vi "Analytical Inverse Kinematics (6R Type 1).vi"(8 "error in (no error)":errorcluster, 10 "end effector transform":T1, 11 "6R type 1 serial arm in":refnum<class "NI_Robotics_6R Type 1 Serial Arm Class.lvclass">) -> (0 "error out":errorcluster, 1 "number of valid solutions":i32, 2 "joint positions":T1, 3 "6R type 1 serial arm out":refnum<class "NI_Robotics_6R Type 1 Serial Arm Class.lvclass">)   [LabVIEW 2017, in "NI_Robotics_6R Type 1 Serial Arm Class.lvclass"]
doc: "Returns the joint angles of a 6R, 5R, or SCARA arm given the posture of the end effector relative to the arm base. Wire data to the <B>X</B><B>_serial arm in</B> input, where <B>X</B> is the arm type, to determine the polymorphic instance to use or manually select the instance."
uses:
  <vilib>/robotics/Kinematics/Analytical/6R/Type 1/NI_Robotics_6R Type 1 Serial Arm Class.lvclass
  c:/Program Files (x86)/National Instruments/LabVIEW 2017/vi.lib/robotics/Kinematics/Robot/NI_Robotics_Serial Robot Arm.lvclass
  c:/Program Files (x86)/National Instruments/LabVIEW 2017/vi.lib/robotics/Kinematics/Analytical/Generic/NI_Robotics_Analytical Serial Arm Class.lvclass
  <vilib>/Analysis/Matrix/Datatypes/RealMatrix.ctl
  <vilib>/robotics/Kinematics/Link/NI_Robotics_Link.lvclass/NI_Robotics_Link.ctl
  <vilib>/Analysis/baseanly.llb/Real A x B.vi
  <vilib>/robotics/Kinematics/Link/Get Kinematic Parameters.vi
  <vilib>/robotics/Kinematics/Analytical/Generic/NI_Robotics_Analytical Serial Arm Class.lvclass
  <vilib>/robotics/Kinematics/Analytical/Generic/Accessors/Read alpha_n0.vi
  <vilib>/robotics/Kinematics/Robot/Get Links.vi
  <vilib>/Analysis/baseanly.llb/Real Inverse Matrix.vi
  <vilib>/robotics/Kinematics/Robot/NI_Robotics_Serial Robot Arm.lvclass
  <vilib>/Analysis/NI_AALBase.lvlib
  <vilib>/robotics/Kinematics/NI_Kinematics.lvlib
  <vilib>/Analysis/Matrix/NI_Matrix.lvlib
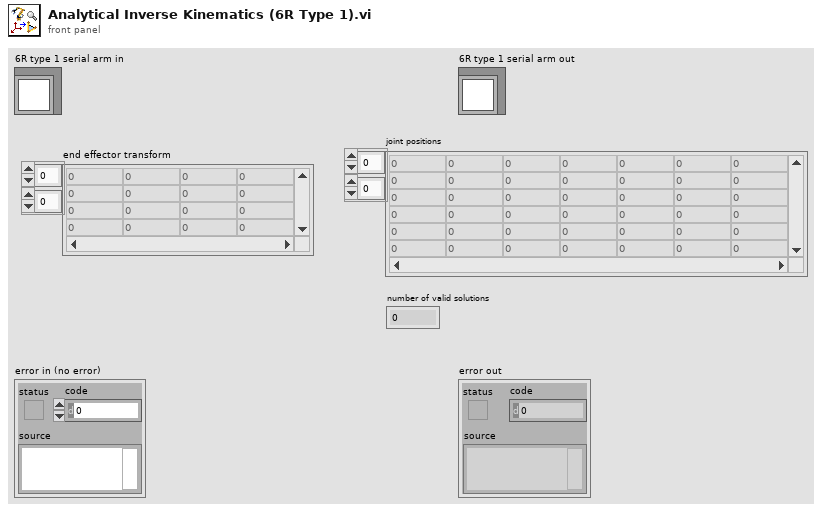
[diagram p1: front panel]
types:
  T1 = typedef "NI_Matrix.lvlib/RealMatrix.ctl" = dbl[][]
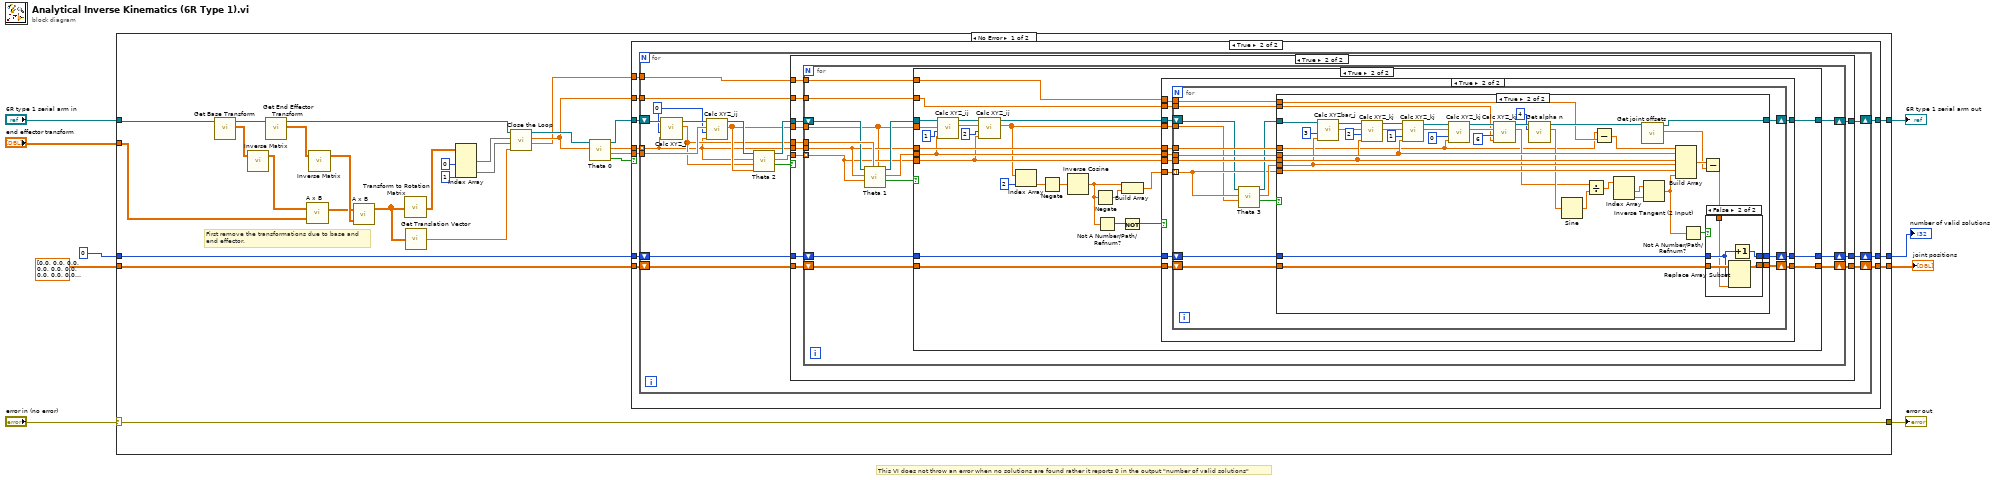
[diagram p0: block diagram]
diagram:
  # "This VI does not throw an error when no solutions are found rather it reports 0 in the output \"number of valid solutions\""
  n1 = case shown="No Error" "error in (no error)" {
    selector: "error in (no error)" -> [w38 w215]
    tunnel: [w38 w215] -> w8
    tunnel: [w27 w214] -> w6
    tunnel: "6R type 1 serial arm in" -> [w18 w214]
    tunnel: "end effector transform" -> [w12 _]
    tunnel: dbl[][] [[0.0, 0.0, 0.0, 0.0, 0.0, 0.0], [0.0, 0.0, 0.0, 0.0, 0.0, 0.0], [0.0, 0.0, 0.0, 0.0, 0.0, 0.0], [0.0, 0.0, 0.0, 0.0, 0.0, 0.0], [0.0, 0.0, 0.0, 0.0, 0.0, 0.0], [0.0, 0.0, 0.0, 0.0, 0.0, 0.0], [0.0, 0.0, 0.0, 0.0, 0.0, 0.0], [0.0, 0.0, 0.0, 0.0, 0.0, 0.0]] ("Solutions") -> [w26 w212]
    tunnel: [w25 w212] -> w1
    tunnel: 0 -> [w24 w213]
    tunnel: [w23 w213] -> w2
    frame No Error {
      # "First remove the transformations due to base and\nend effector."
      n2 = call <vilib>:"Get Base Transform.vi"("serial arm in"=w18) -> ("base transform"=w35:T1, "serial arm out"=w37:refnum<class "NI_Robotics_6R Type 1 Serial Arm Class.lvclass">)  [unwired: 8 in, 1 out]
      n3 = call-poly <vilib>:"Inverse Matrix.vi"("Input Matrix"=w35) -> ("Inverse Matrix"=w13:T1)  [unwired: 1 in, 1 out]
      n4 = call <vilib>:"Get End Effector Transform.vi"("serial arm in"=w37) -> ("end effector transform"=w36:T1, "serial arm out"=w30:refnum<class "NI_Robotics_6R Type 1 Serial Arm Class.lvclass">)  [unwired: 8 in, 1 out]
      n5 = call-poly <vilib>:"A x B.vi"("B"=w12, "A"=w13) -> ("A x B"=w10:T1)  [unwired: 1 out]
      n6 = call-poly <vilib>:"Inverse Matrix.vi"("Input Matrix"=w36) -> ("Inverse Matrix"=w11:T1)  [unwired: 1 in, 1 out]
      n7 = call-poly <vilib>:"A x B.vi"("B"=w11, "A"=w10) -> ("A x B"=w34:T1)  [unwired: 1 out]
      n8 = call <vilib>:"Transform to Rotation Matrix.vi"("transform"=w34) -> ("rotation matrix"=w20:T1)
      n9 = call <vilib>:"Get Translation Vector.vi"("transform"=w34) -> ("translation vector"=w29:dbl[])
      n10 = Index Array(array=w20, index (col) #1=0 ("disabled index (col)"), index (col) #2=1 ("index (col)")) -> (element #1=w17:dbl[], element #2=w19:dbl[])  [unwired: 2 in]
      n11 = call <vilib>:"Close the Loop.vi"("P_toolf"=w29, "S_n-1f"=w19, "a_(n-1)nf"=w17, "Analytical Serial Arm Class in"=w30) -> ("gamma_0"=w14:dbl, "theta_n"=w15:dbl, "Analytical Serial Arm Class out"=w16:refnum<class "NI_Robotics_6R Type 1 Serial Arm Class.lvclass">)  [unwired: 5 in]
      n12 = call <vilib>:"Theta 0.vi"("theta_6"=w15, "6R Type 1 Serial Arm Class in"=w16) -> ("Valid?"=w28:bool, "XYZ_6"=w32:dbl[], "theta_0 array"=w33:dbl[], "6R Type 1 Serial Arm Class out"=w31:refnum<class "NI_Robotics_6R Type 1 Serial Arm Class.lvclass">)  [unwired: 6 in]
      n13 = case shown="True" w28 {
        tunnel: w33 -> [_ w51]
        tunnel: w32 -> [_ w50]
        tunnel: w31 -> [w41 w49]
        tunnel: [w41 w48] -> w27
        tunnel: w15 -> [_ w47]
        tunnel: w26 -> [w39 w46]
        tunnel: [w39 w45] -> w25
        tunnel: w24 -> [w40 w44]
        tunnel: [w40 w43] -> w23
        tunnel: w14 -> [_ w42]
        frame False {
        }
        frame True {
          n14 = for {
            tunnel: w51 -> [w60] mode=indexing
            tunnel: w50 -> [w67]
            shift-right: [w58] -> w48
            shift-left: w49 -> [w69]
            tunnel: w47 -> [w57]
            shift-right: [w55] -> w45
            shift-left: w46 -> [w56]
            shift-right: [w53] -> w43
            shift-left: w44 -> [w54]
            tunnel: w42 -> [w52]
            w66 = 0 ("j")
            n15 = call <vilib>:"Calc XYZ_j.vi"("theta_j"=w60, "j"=w66, "Analytical Serial Arm Class in"=w69) -> ("XYZ_j"=w61:dbl[], "Analytical Serial Arm Class out"=w68:refnum<class "NI_Robotics_6R Type 1 Serial Arm Class.lvclass">)  [unwired: 7 in]
            n16 = call <vilib>:"Calc XYZ_ij.vi"("theta_j"=w60, "j"=w66, "XYZ_i"=w67, "Analytical Serial Arm Class in"=w68) -> ("XYZ_ij"=w62:dbl[], "Analytical Serial Arm Class out"=w65:refnum<class "NI_Robotics_6R Type 1 Serial Arm Class.lvclass">)  [unwired: 5 in, 1 out]
            n17 = call <vilib>:"Theta 2.vi"("XYZ_60"=w62, "XYZ_0"=w61, "theta_0"=w60, "6R Type 1 Serial Arm Class in"=w65) -> ("Valid"=w59:bool, "theta_2 array"=w64:dbl[], "6R Type 1 Serial Arm Class out"=w63:refnum<class "NI_Robotics_6R Type 1 Serial Arm Class.lvclass">)  [unwired: 5 in]
            n18 = case shown="True" w59 {
              tunnel: w64 -> [_ w84]
              tunnel: w63 -> [w72 w83]
              tunnel: w62 -> [_ w82]
              tunnel: w61 -> [_ w81]
              tunnel: w60 -> [_ w80]
              tunnel: [w72 w79] -> w58
              tunnel: w57 -> [_ w78]
              tunnel: w56 -> [w70 w77]
              tunnel: [w70 w76] -> w55
              tunnel: w54 -> [w71 w75]
              tunnel: [w71 w74] -> w53
              tunnel: w52 -> [_ w73]
              frame False {
              }
              frame True {
                n19 = for {
                  tunnel: w84 -> [w93] mode=indexing
                  tunnel: w82 -> [w92]
                  tunnel: w81 -> [w99]
                  tunnel: w80 -> [w94]
                  shift-right: [w91] -> w79
                  shift-left: w83 -> [w98]
                  tunnel: w78 -> [w90]
                  shift-right: [w88] -> w76
                  shift-left: w77 -> [w89]
                  shift-right: [w86] -> w74
                  shift-left: w75 -> [w87]
                  tunnel: w73 -> [w85]
                  n20 = call <vilib>:"Theta 1.vi"("XYZ_60"=w92, "XYZ_0"=w99, "theta 2"=w93, "theta 0"=w94, "6R Type 1 Serial Arm Class in"=w98) -> ("Valid"=w96:bool, "theta 1"=w95:dbl, "6R Type 1 Serial Arm Class out"=w97:refnum<class "NI_Robotics_6R Type 1 Serial Arm Class.lvclass">)  [unwired: 4 in]
                  n21 = case shown="True" w96 {
                    tunnel: w97 -> [w102 w128]
                    tunnel: w95 -> [_ w113]
                    tunnel: w94 -> [_ w114]
                    tunnel: w93 -> [_ w112]
                    tunnel: w92 -> [_ w127]
                    tunnel: [w102 w110] -> w91
                    tunnel: w90 -> [_ w108]
                    tunnel: w89 -> [w100 w107]
                    tunnel: [w100 w106] -> w88
                    tunnel: w87 -> [w101 w105]
                    tunnel: [w101 w104] -> w86
                    tunnel: w85 -> [_ w103]
                    frame False {
                    }
                    frame True {
                      n22 = call <vilib>:"Calc XYZ_ij.vi"("theta_j"=w113, "j"=1, "XYZ_i"=w127, "Analytical Serial Arm Class in"=w128) -> ("XYZ_ij"=w125:dbl[], "Analytical Serial Arm Class out"=w124:refnum<class "NI_Robotics_6R Type 1 Serial Arm Class.lvclass">)  [unwired: 5 in, 1 out]
                      n23 = call <vilib>:"Calc XYZ_ij.vi"("theta_j"=w112, "j"=2, "XYZ_i"=w125, "Analytical Serial Arm Class in"=w124) -> ("XYZ_ij"=w109:dbl[], "Analytical Serial Arm Class out"=w111:refnum<class "NI_Robotics_6R Type 1 Serial Arm Class.lvclass">)  [unwired: 5 in, 1 out]
                      n24 = Index Array(array=w109, index=2) -> (element=w121:dbl)
                      n25 = Negate(x=w121) -> (-x=w120:dbl)
                      n26 = Inverse Cosine(1:w120) -> (0:w118:dbl)
                      n27 = Negate(x=w118) -> (-x=w119:dbl)
                      n28 = Not A Number/Path/Refnum?(number/path/refnum=w118) -> (NaN/Path/Refnum?=w117:bool)
                      n29 = Not(x=w117) -> (.not. x?=w116:bool)
                      n30 = Build Array(w118, w119) -> (w115:dbl[])
                      n31 = case shown="True" w116 {
                        tunnel: w115 -> [_ w144]
                        tunnel: w114 -> [_ w140]
                        tunnel: w113 -> [_ w139]
                        tunnel: w112 -> [_ w138]
                        tunnel: w111 -> [w131 w143]
                        tunnel: [w131 w142] -> w110
                        tunnel: w109 -> [_ w141]
                        tunnel: w108 -> [_ w137]
                        tunnel: w107 -> [w129 w136]
                        tunnel: [w129 w135] -> w106
                        tunnel: w105 -> [w130 w134]
                        tunnel: [w130 w133] -> w104
                        tunnel: w103 -> [_ w132]
                        frame False {
                        }
                        frame True {
                          n32 = for {
                            tunnel: w144 -> [w154] mode=indexing
                            shift-right: [w152] -> w142
                            shift-left: w143 -> [w146]
                            tunnel: w141 -> [w145]
                            tunnel: w140 -> [w159]
                            tunnel: w139 -> [w158]
                            tunnel: w138 -> [w157]
                            tunnel: w137 -> [w153]
                            shift-right: [w150] -> w135
                            shift-left: w136 -> [w151]
                            shift-right: [w148] -> w133
                            shift-left: w134 -> [w149]
                            tunnel: w132 -> [w147]
                            n33 = call <vilib>:"Theta 3.vi"("XYZ_ij"=w145, "theta_4"=w154, "6R Type 1 Serial Arm Class in"=w146) -> ("valid?"=w160:bool, "theta_3"=w155:dbl, "6R Type 1 Serial Arm Class out"=w156:refnum<class "NI_Robotics_6R Type 1 Serial Arm Class.lvclass">)  [unwired: 6 in]
                            n34 = case shown="True" w160 {
                              tunnel: w159 -> [_ w165]
                              tunnel: w158 -> [_ w187]
                              tunnel: w157 -> [_ w186]
                              tunnel: w156 -> [w163 w204]
                              tunnel: w155 -> [_ w185]
                              tunnel: w154 -> [_ w184]
                              tunnel: w153 -> [_ w190]
                              tunnel: [w163 w177] -> w152
                              tunnel: w151 -> [w161 w183]
                              tunnel: [w161 w182] -> w150
                              tunnel: w149 -> [w162 w181]
                              tunnel: [w162 w180] -> w148
                              tunnel: w147 -> [_ w166]
                              frame False {
                              }
                              frame True {
                                n35 = call <vilib>:"Calc XYZbar_j.vi"("theta_j"=w185, "j"=3, "Analytical Serial Arm Class in"=w204) -> ("XYZbar_j"=w201:dbl[], "Analytical Serial Arm Class out"=w202:refnum<class "NI_Robotics_6R Type 1 Serial Arm Class.lvclass">)  [unwired: 7 in]
                                n36 = call <vilib>:"Calc XYZ_kj.vi"("theta_j"=w186, "j"=2, "XYZbar_k"=w201, "Analytical Serial Arm Class in"=w202) -> ("XYZ_ij"=w198:dbl[], "Analytical Serial Arm Class out"=w199:refnum<class "NI_Robotics_6R Type 1 Serial Arm Class.lvclass">)  [unwired: 5 in, 1 out]
                                n37 = call <vilib>:"Calc XYZ_kj.vi"("theta_j"=w187, "j"=1, "XYZbar_k"=w198, "Analytical Serial Arm Class in"=w199) -> ("XYZ_ij"=w194:dbl[], "Analytical Serial Arm Class out"=w196:refnum<class "NI_Robotics_6R Type 1 Serial Arm Class.lvclass">)  [unwired: 5 in, 1 out]
                                n38 = call <vilib>:"Calc XYZ_kj.vi"("theta_j"=w165, "j"=0, "XYZbar_k"=w194, "Analytical Serial Arm Class in"=w196) -> ("XYZ_ij"=w192:dbl[], "Analytical Serial Arm Class out"=w193:refnum<class "NI_Robotics_6R Type 1 Serial Arm Class.lvclass">)  [unwired: 5 in, 1 out]
                                n39 = call <vilib>:"Calc XYZ_kj.vi"("theta_j"=w190, "j"=6, "XYZbar_k"=w192, "Analytical Serial Arm Class in"=w193) -> ("XYZ_ij"=w169:dbl[], "Analytical Serial Arm Class out"=w173:refnum<class "NI_Robotics_6R Type 1 Serial Arm Class.lvclass">)  [unwired: 5 in, 1 out]
                                n40 = call <vilib>:"Get alpha n.vi"("n"=4, "Analytical Serial Arm Class in"=w173) -> ("alpha n"=w170:dbl, "Analytical Serial Arm Class out"=w172:refnum<class "NI_Robotics_6R Type 1 Serial Arm Class.lvclass">)  [unwired: 8 in]
                                n41 = Sine(x=w170) -> (sin(x)=w168:dbl)
                                n42 = Divide(x=w169, y=w168) -> (x/y=w167:dbl[])
                                n43 = Subtract(x=w165, y=w166) -> (x-y=w164:dbl)
                                n44 = Index Array(array=w167) -> (element #1=w189:dbl, element #2=w188:dbl)  [unwired: 2 in]
                                n45 = call <vilib>:"Get joint offsets.vi"("Analytical Serial Arm Class in"=w172) -> ("joint offsets"=w175:dbl[], "Analytical Serial Arm Class out"=w177:refnum<class "NI_Robotics_6R Type 1 Serial Arm Class.lvclass">)  [unwired: 9 in]
                                n46 = Inverse Tangent (2 Input)(1:w188, 2:w189) -> (0:w178:dbl)
                                n47 = Build Array(w164, w187, w186, w185, w184, w178) -> (w176:dbl[])
                                n48 = Not A Number/Path/Refnum?(number/path/refnum=w178) -> (NaN/Path/Refnum?=w179:bool)
                                n49 = Subtract(x=w176, y=w175) -> (x-y=w174:dbl[])
                                n50 = case shown="False" w179 {
                                tunnel: w183 -> [w205 w211]
                                tunnel: [w205 w210] -> w182
                                tunnel: w181 -> [w206 w209]
                                tunnel: [w206 w208] -> w180
                                tunnel: w174 -> [_ w207]
                                frame True {
                                }
                                frame False {
                                n51 = Replace Array Subset(array=w211, new element=w207, index (row)=w209) -> (w210:dbl[][])  [unwired: 1 in]
                                n52 = Increment(x=w209) -> (x+1=w208:i32)
                                }
                                }
                              }
                            }
                          }
                        }
                      }
                    }
                  }
                }
              }
            }
          }
        }
      }
    }
    frame Error {
    }
  }
  "error out" <- w8
  "6R type 1 serial arm out" <- w6
  "joint positions" <- w1
  "number of valid solutions" <- w2
